vi "Create ComboBox of ClassNames(冲突时的文件备份2013-03-27 14-06-50).vi"() -> (3 "ClassName":string(combo))   [LabVIEW 2012, in "Application.lvlib"]
uses:
  Application.lvlib
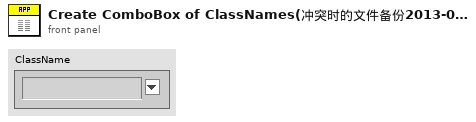
[diagram p1: front panel]
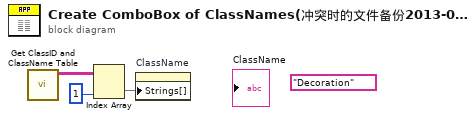
[diagram p0: block diagram]
diagram:
  (unwired) "Decoration" ("ClassName")
  n1 = call "Get ClassID and ClassName Table.vi"() -> ("ClassID and ClassName"=w1:string[][])  [unwired: 10 in, 1 out]
  n2 = Index Array(array=w1, index (col)=1 ("禁用的索引 (列)")) -> (element=w3:string[])  [unwired: 1 in]
  n3 = property on="ClassName" class="CmbBox"("Strings[]"=w3) -> ()  [unwired: 2 in, 2 out]
